vi "RW IMG Attributes.vi"() -> (0 "ErrOut":errorcluster)   [LabVIEW 2014]
doc: "Use this template to build a VI to use as a subVI."
uses:
  <vilib>/vision/NI_Vision_Development_Module.lvlib
panel:
  out "ImageOut":T1(plugin-control)
  in  "ErrIn":errorcluster
  # "Input Parameters"
  # "Output Parameters"
  # "VI Description:\nThis VI is .."
  # ":: MVI Framework V1.0 ::\nAuthor:Gaoke Yang\nEmail: gaoke.yang@yahoo.com\nWeb: www.mvicontrol.com\nCopyright (C) 2013, MVI Technologies All Rights Reserved"
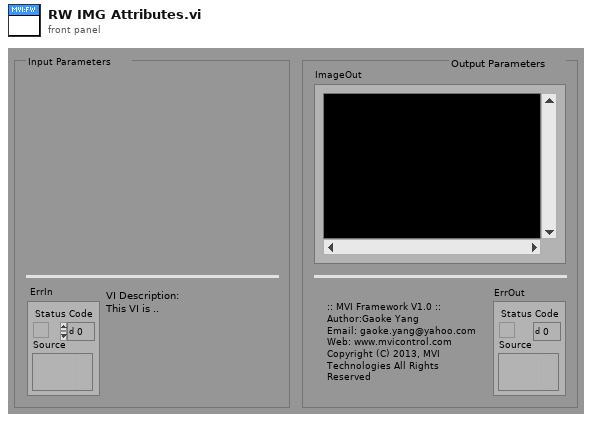
[diagram p1: front panel]
types:
  T1 = typedef "IMAQ Image.ctl" = refnum<image>
  T2 = typedef "Image Type" = u32
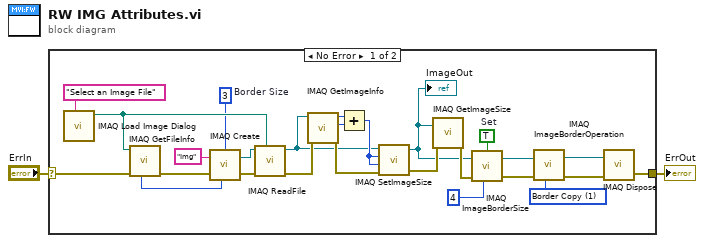
[diagram p0: block diagram]
diagram:
  n1 = case shown="No Error" "ErrIn" {
    selector: "ErrIn" -> [w23 w29]
    tunnel: [w22 w29] -> w2
    frame No Error {
      w3 = u32 1 items=["Border Mirror", "Border Copy", "Border Clear"] ("Function")
      w16 = TRUE  # Set
      w19 = 3  # Border Size
      n2 = call "IMAQ Load Image Dialog"("Prompt"="Select an Image File" ("prompt")) -> ("Path"=w21:path)  [unwired: 8 in, 2 out]
      n3 = call "IMAQ GetFileInfo"("error in (no error)"=w23, "File Path"=w21) -> ("error out"=w24:errorcluster, "Image Type"=w20:T2)  [unwired: 3 in, 5 out]
      n4 = call "IMAQ Create"("Border Size"=w19, "Image Name"="Img", "Image Type"=w20, "error in (no error)"=w24) -> ("New Image"=w27:T1, "error out"=w26:errorcluster)  [unwired: 1 in]
      n5 = call "IMAQ ReadFile"("File Path"=w21, "error in (no error)"=w26, "Image"=w27) -> ("error out"=w5:errorcluster, "Image Out"=w4:T1)  [unwired: 4 in, 3 out]
      n6 = call "IMAQ GetImageInfo"("error in (no error)"=w5, "Image"=w4) -> ("error out"=w15:errorcluster, "Y Resolution"=w13:i32, "X Resolution"=w14:i32)  [unwired: 2 in, 5 out]
      n7 = Add(x=w14, y=w13) -> (x+y=w12:i32)
      n8 = call "IMAQ SetImageSize"("error in (no error)"=w15, "Y Resolution"=w12, "X Resolution"=w12, "Image"=w4) -> ("error out"=w11:errorcluster, "Image Out"=w6:T1)  [unwired: 1 in]
      "ImageOut" <- w6
      n9 = call "IMAQ GetImageSize"("Image"=w6, "error in (no error)"=w11) -> ("error out"=w7:errorcluster)  [unwired: 2 in, 2 out]
      n10 = call "IMAQ ImageBorderSize"("Get/Set Status? (Set)"=w16, "Image"=w6, "Image border size in"=4, "error in (no error)"=w7) -> ("Image Out"=w8:T1, "error out"=w9:errorcluster)  [unwired: 1 out]
      n11 = call "IMAQ ImageBorderOperation"("Image"=w8, "Function"=w3, "error in (no error)"=w9) -> ("Image Out"=w18:T1, "error out"=w17:errorcluster)  [unwired: 2 in]
      n12 = call "IMAQ Dispose"("Image"=w18, "error in (no error)"=w17) -> ("error out"=w22:errorcluster)  [unwired: 4 in]
    }
    frame Error {
    }
  }
  "ErrOut" <- w2
